vi "PID DAQ Save.vi"(6 "Sample Parameter Names":string[](array[string]), 7 "Sample Data":dbl[][](array[numeric]), 8 "error in":errorcluster, 9 "Sample Name":string, 10 "Sample Parameters":variant[](array[variant]), 11 "TDMS in":refnum<class "TDMS.lvclass">) -> (0 "error out":errorcluster, 3 "TDMS out":refnum<class "TDMS.lvclass">)   [LabVIEW 2011]
uses:
  Modules/File/TDMS/TDMS.lvclass
  Modules/File/TDMS/File Level.ctl
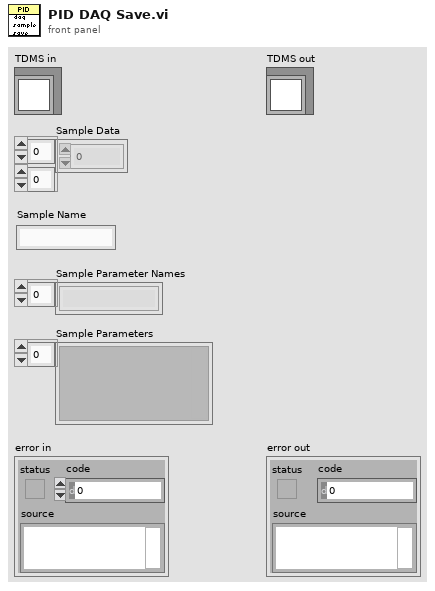
[diagram p1: front panel]
types:
  T1 = typedef "TDMS.lvclass/File Level.ctl" = enum16{"File", "Group", "Channel"}
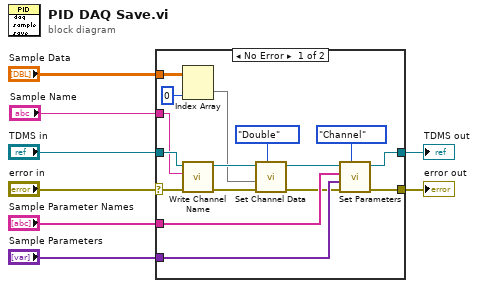
[diagram p0: block diagram]
diagram:
  n1 = case shown="No Error" "error in" {
    selector: "error in" -> [w14 w25]
    tunnel: "Sample Parameters" -> [w24 _]
    tunnel: "Sample Parameter Names" -> [w23 _]
    tunnel: [w22 w25] -> w6
    tunnel: [w21 w26] -> w5
    tunnel: "Sample Data" -> [w11 _]
    tunnel: "TDMS in" -> [w15 w26]
    tunnel: "Sample Name" -> [w12 _]
    frame No Error {
      n2 = Index Array(array=w11, index (col)=0 ("disabled index (col)")) -> (element=w10:dbl[])  [unwired: 1 in]
      n3 = call-dynamic "Write Channel Name.vi"("error in (no error)"=w14, "Channel Name"=w12, "TDMS in"=w15) -> ("error out"=w20:errorcluster, "TDMS out"=w17:refnum<class "TDMS.lvclass">)  [unwired: 7 in]
      n4 = call-dynamic "Set Channel Data.vi"("data type"=enum16{"I16", "Double"}."Double" ("Data Type"), "error in"=w20, "double channel data"=w10, "TDMS in"=w17) -> ("error out"=w13:errorcluster, "TDMS out"=w18:refnum<class "TDMS.lvclass">)  [unwired: 6 in]
      n5 = call-dynamic "Set Parameters.vi"("File Level"=File_Level."Channel", "error in (no error)"=w13, "property values"=w24, "property names"=w23, "TDMS.lvclass in"=w18) -> ("error out"=w22:errorcluster, "TDMS.lvclass out"=w21:refnum<class "TDMS.lvclass">)  [unwired: 5 in]
    }
    frame Error {
    }
  }
  "error out" <- w6
  "TDMS out" <- w5
